vi "picoquant_write_metadata.vi"(8 "error in (no error)":errorcluster, 11 "hydraharp in":refnum<class "hydraharp.lvclass">) -> (0 "error out":errorcluster, 3 "hydraharp out":refnum<class "hydraharp.lvclass">)   [LabVIEW 2015, in "hydraharp.lvclass"]
uses:
  hydraharp.lvclass
  hydraharp.lvclass/hydraharp.ctl
  hdf5_photon_record_logger/stream_metadata.ctl
  hydraharp_panel/hpanel_hydraharp_settings.ctl
  hydraharp_panel/hpanel_sync_settings.ctl
  hydraharp_panel/hpanel_sync_div.ctl
  hydraharp_panel/hpanel_channel_settings.ctl
  Data Logger Class/data_logger.lvclass
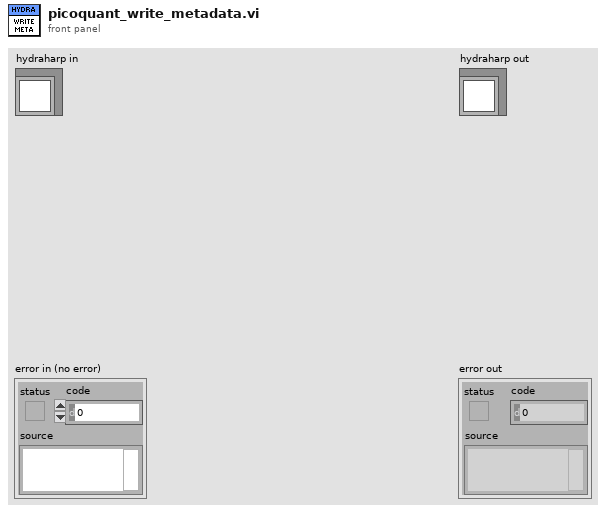
[diagram p1: front panel]
types:
  T1 = typedef "stream_metadata.ctl" = cluster{"Hydraharp Settings":T2, "resolution":dbl, "stream_notes":string}
  T2 = typedef "hpanel_hydraharp_settings.ctl" = cluster{"Sync Settings":T3, "CH 1":T5, "CH 2":T5, "CH 3":T5, "CH 4":T5, "binning":i32, "CH 5":T5, "CH 6":T5, "CH 7":T5, "CH 8":T5}
  T3 = typedef "hpanel_sync_settings.ctl" = cluster{"snc_count":i32, "snc_level":i32, "snc_ZeroX":i32, "snc_offs":i32, "sync_div":T4}
  T4 = typedef "hpanel_sync_div.ctl" = enum16{"1", "2", "4", "8"}
  T5 = typedef "hpanel_channel_settings.ctl" = cluster{"ch_counts":i32, "ch_level":i32, "ch_ZeroX":i32, "ch_offs":i32}
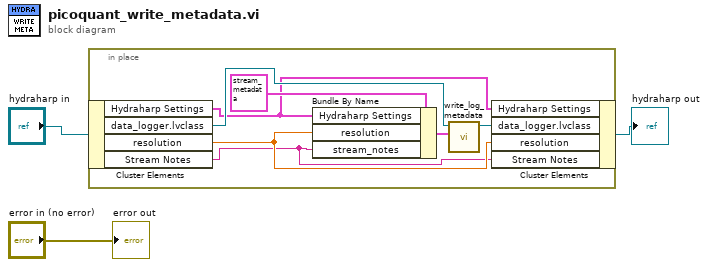
[diagram p0: block diagram]
diagram:
  n1 = in-place {
    n2 = in-place-cluster #1("hydraharp in") -> ("Hydraharp Settings"=w6:T2, "data_logger.lvclass"=w8:refnum<class "data_logger.lvclass">, "resolution"=w5:dbl, "Stream Notes"=w4:string)
    n3 = Bundle By Name(cluster=T1 {"Hydraharp Settings"={"Sync Settings"={"snc_count"=0, "snc_level"=0, "snc_ZeroX"=0, "snc_offs"=0, "sync_div"=enum."1"}, "CH 1"={"ch_counts"=0, "ch_level"=0, "ch_ZeroX"=0, "ch_offs"=0}, "CH 2"={"ch_counts"=0, "ch_level"=0, "ch_ZeroX"=0, "ch_offs"=0}, "CH 3"={"ch_counts"=0, "ch_level"=0, "ch_ZeroX"=0, "ch_offs"=0}, "CH 4"={"ch_counts"=0, "ch_level"=0, "ch_ZeroX"=0, "ch_offs"=0}, "binning"=0, "CH 5"={"ch_counts"=0, "ch_level"=0, "ch_ZeroX"=0, "ch_offs"=0}, "CH 6"={"ch_counts"=0, "ch_level"=0, "ch_ZeroX"=0, "ch_offs"=0}, "CH 7"={"ch_counts"=0, "ch_level"=0, "ch_ZeroX"=0, "ch_offs"=0}, "CH 8"={"ch_counts"=0, "ch_level"=0, "ch_ZeroX"=0, "ch_offs"=0}}, "resolution"=0.0, "stream_notes"="stream_notes"} ("output cluster"), "Hydraharp Settings"=w6, "resolution"=w5, "stream_notes"=w4) -> (w9:T1)
    n4 = call-dynamic "write_log_metadata.vi"("data"=w9, "data_logger in"=w8) -> ("data_logger out"=w7:refnum<class "data_logger.lvclass">)  [unwired: 8 in, 1 out]
    n5 = in-place-cluster #1("Hydraharp Settings"=w6, "data_logger.lvclass"=w7, "resolution"=w5, "Stream Notes"=w4) -> (→"hydraharp out":refnum<class "hydraharp.lvclass">)
  }
  "error out" <- "error in (no error)"
